vi "Resize Listbox Columns.vi"(5 "[user-specified font]":T2, 7 "desired font(Application)":T1(ring)=enum."Application Font", 8 "error in (no error)":errorcluster, 9 "Max Width (300px)":i16=300, 10 "Padding (5px)":i16=5, 11 "Listbox Control ref in":refnum<vi>) -> (0 "error out":errorcluster, 3 "Listbox Control ref out":refnum<vi>)   [LabVIEW 2013, in "SET Project Editor.lvlib"]
doc: "Resize Listbox Columns.vi\n\nResizes MCLB columns based on cell contents.\n\nOptions\nPadding (5px): Cell padding in pixels\nMax Width (300px): Maximum column width\ndesired font(Application) & [user-specified-font]: Assumed font of MCLB contents."
uses:
  SET Project Editor.lvlib
  <vilib>/Utility/miscctls.llb/LVRowAndColumnTypeDef.ctl
panel:
  # "Resize Listbox Columns.vi\n\nResizes MCLB columns based on cell contents.\n\nOptions\nPadding (5px): Cell padding in pixels\nMax Width (300px): Maximum column width\ndesired font(Application) & [user-specified-font]: Assumed font of MCLB contents."
  # "License: BSD (2-Clause) - http://opensource.org/licenses/BSD-2-Clause \n\nCopyright (c) 2014, Ryan Porter\nAll rights reserved."
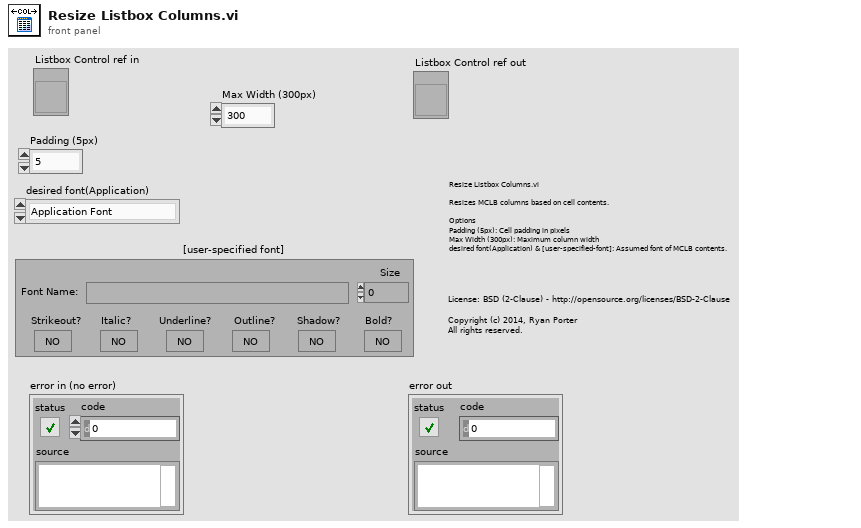
[diagram p1: front panel]
types:
  T1 = enum16{"User-specified Font", "Application Font", "System Font", "Dialog Font"}
  T2 = cluster{"Font Name:":string, "Size":i16, "Strikeout?":bool, "Italic?":bool, "Underline?":bool, "Outline?":bool, "Shadow?":bool, "Bold?":bool}
  T3 = typedef "LVRowAndColumnTypeDef.ctl" = cluster{"Row":i32, "Column":i32}
  T4 = cluster{"left":i16, "top":i16, "right":i16, "bottom":i16}
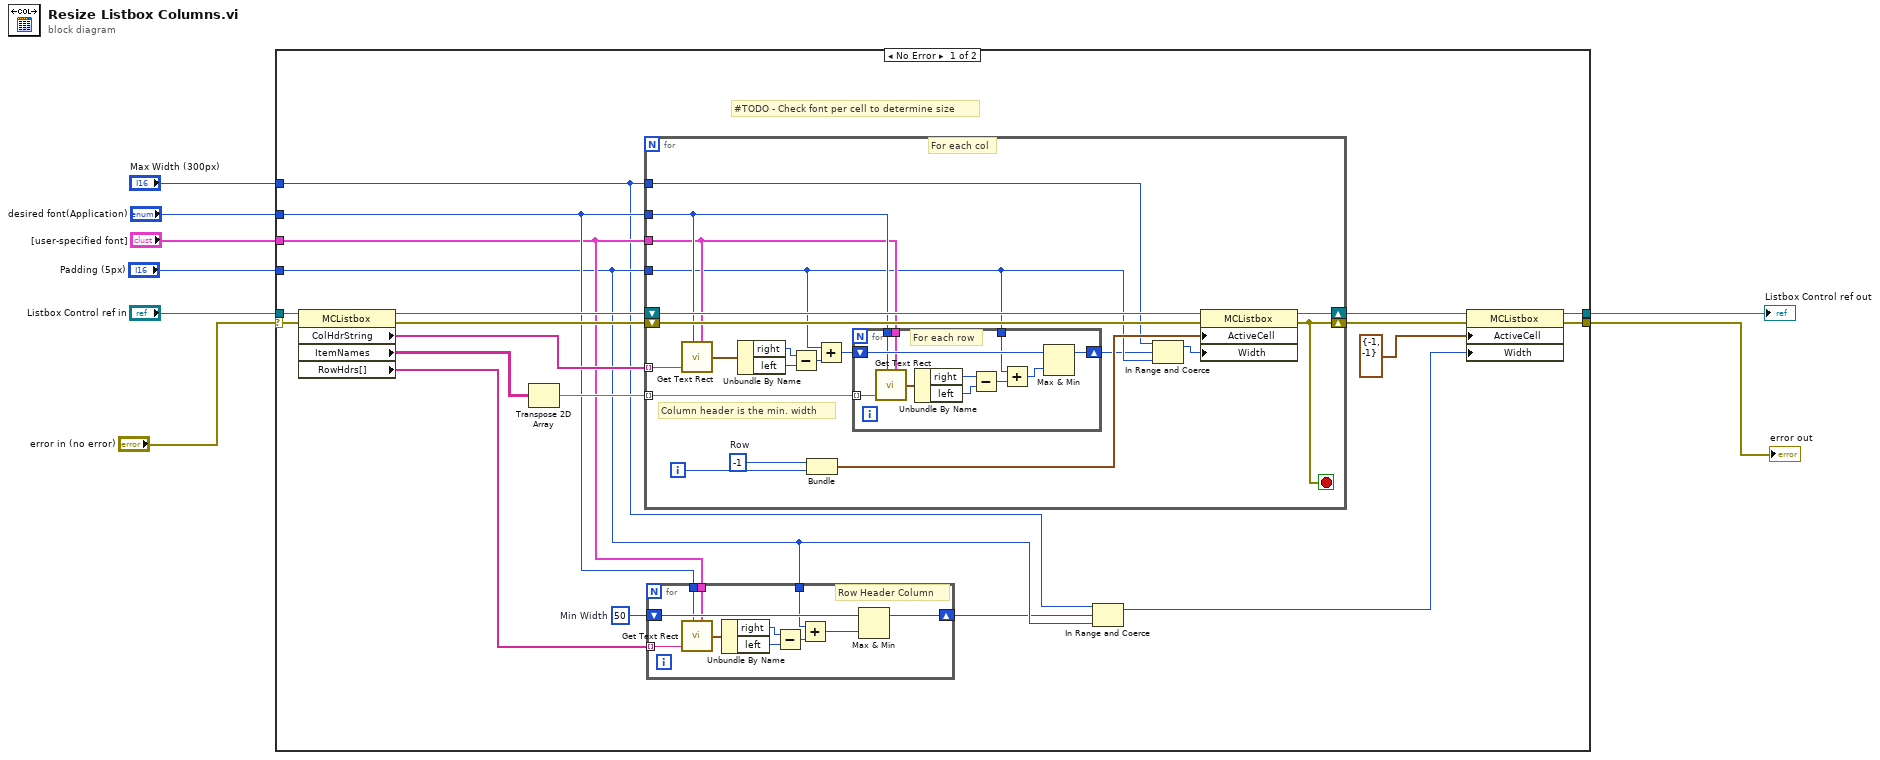
[diagram p0: block diagram]
diagram:
  n1 = case shown="No Error" "error in (no error)" {
    selector: "error in (no error)" -> [w22 w71]
    tunnel: "Listbox Control ref in" -> [w28 w72]
    tunnel: "Padding (5px)" -> [w12 _]
    tunnel: [w17 w72] -> w7
    tunnel: [w15 w71] -> w6
    tunnel: "desired font(Application)" -> [w14 _]
    tunnel: "[user-specified font]" -> [w13 _]
    tunnel: "Max Width (300px)" -> [w11 _]
    frame No Error {
      w20 = i16 50  # Min Width
      # "#TODO - Check font per cell to determine size"
      n2 = property class="MCListbox"(reference=w28, error in=w22) -> (reference out=w24:refnum<vi>, error out=w23:errorcluster, "ColHdrString"=w25:string[], "ItemNames"=w27:string[][], "RowHdrs[]"=w21:string[])
      n3 = Transpose 2D Array(2D array=w27) -> (transposed array=w26:string[][])
      n4 = for {
        tunnel: w26 -> [w59] mode=indexing
        tunnel: w25 -> [w58] mode=indexing
        tunnel: w12 -> [w42]
        shift-right: [w49] -> w16
        shift-left: w23 -> [w50]
        tunnel: w14 -> [w45]
        tunnel: w13 -> [w44]
        tunnel: w11 -> [w43]
        shift-right: [w51] -> w18
        shift-left: w24 -> [w52]
        i -> [w55]
        stop <- w49 stop-if-true
        w54 = -1  # Row
        # "For each col"
        # "Column header is the min. width"
        n5 = call <vilib>:"Get Text Rect.vi"("desired font(Application)"=w45, "text"=w58, "[user-specified font]"=w44) -> ("rect"=w57:T4)  [unwired: 6 in]
        n6 = Unbundle By Name(w57) -> ("right"=w48:i16, "left"=w47:i16)
        n7 = Subtract(x=w48, y=w47) -> (x-y=w46:i16)
        n8 = Bundle("Row"=w54, w55) -> (w53:cluster{"Row":i32, i32})  [unwired: 1 in]
        n9 = Add(x=w42, y=w46) -> (x+y=w56:i16)
        n10 = for {
          tunnel: w59 -> [w70] mode=indexing
          shift-right: [w67] -> w41
          shift-left: w56 -> [w68]
          tunnel: w42 -> [w63]
          tunnel: w45 -> [w61]
          tunnel: w44 -> [w60]
          # "For each row"
          n11 = call <vilib>:"Get Text Rect.vi"("desired font(Application)"=w61, "text"=w70, "[user-specified font]"=w60) -> ("rect"=w69:T4)  [unwired: 6 in]
          n12 = Unbundle By Name(w69) -> ("right"=w66:i16, "left"=w65:i16)
          n13 = Subtract(x=w66, y=w65) -> (x-y=w64:i16)
          n14 = Add(x=w63, y=w64) -> (x+y=w62:i16)
          n15 = Max & Min(x=w68, y=w62) -> (max(x,y)=w67:i16)  [unwired: 1 out]
        }
        n16 = In Range and Coerce(upper limit=w43, x=w41, lower limit=w42) -> (coerced(x)=w40:i16)  [unwired: 1 out]
        n17 = property class="MCListbox"(reference=w52, error in=w50, "ActiveCell"=w53, "Width"=w40) -> (reference out=w51:refnum<vi>, error out=w49:errorcluster)
      }
      n18 = for {
        tunnel: w21 -> [w35] mode=indexing
        shift-right: [w33] -> w10
        shift-left: w20 -> [w32]
        tunnel: w12 -> [w31]
        tunnel: w14 -> [w30]
        tunnel: w13 -> [w29]
        # "Row Header Column"
        n19 = call <vilib>:"Get Text Rect.vi"("desired font(Application)"=w30, "text"=w35, "[user-specified font]"=w29) -> ("rect"=w36:T4)  [unwired: 6 in]
        n20 = Unbundle By Name(w36) -> ("right"=w37:i16, "left"=w38:i16)
        n21 = Subtract(x=w37, y=w38) -> (x-y=w39:i16)
        n22 = Add(x=w31, y=w39) -> (x+y=w34:i16)
        n23 = Max & Min(x=w32, y=w34) -> (max(x,y)=w33:i16)  [unwired: 1 out]
      }
      n24 = In Range and Coerce(upper limit=w11, x=w10, lower limit=w12) -> (coerced(x)=w9:i16)  [unwired: 1 out]
      n25 = property class="MCListbox"(reference=w18, error in=w16, "ActiveCell"=T3 {"Row"=-1, "Column"=-1} ("Active Cell:Active Cell"), "Width"=w9) -> (reference out=w17:refnum<vi>, error out=w15:errorcluster)
    }
    frame Error {
    }
  }
  "Listbox Control ref out" <- w7
  "error out" <- w6
